vi "test_advanced_Doppler_filtered.vi"() -> ()   [LabVIEW 2009]
doc: "Copyright (C) 2009, Stepan A. Baranov\nweb: http://www.OCTLab.org/\nemail: stepan@baranov.su"
uses:
  OCTLib.dll
panel:
  out "version":string
  out "name":string
  out "error out":errorcluster
  out "max":dbl
  out "min":dbl
  out "window width radius":i32
  out "window height radius":i32
  out "width":i32
  out "height":i32
  in  "Small/Big":bool
  out "loop #":i32
  out "RSM_STAT time":u32
  out "LabView time":u32
  out "RSM_STAT Array":dbl[][](array[numeric])
  out "LabView Array":dbl[][](array[numeric])
  in  "stop":bool
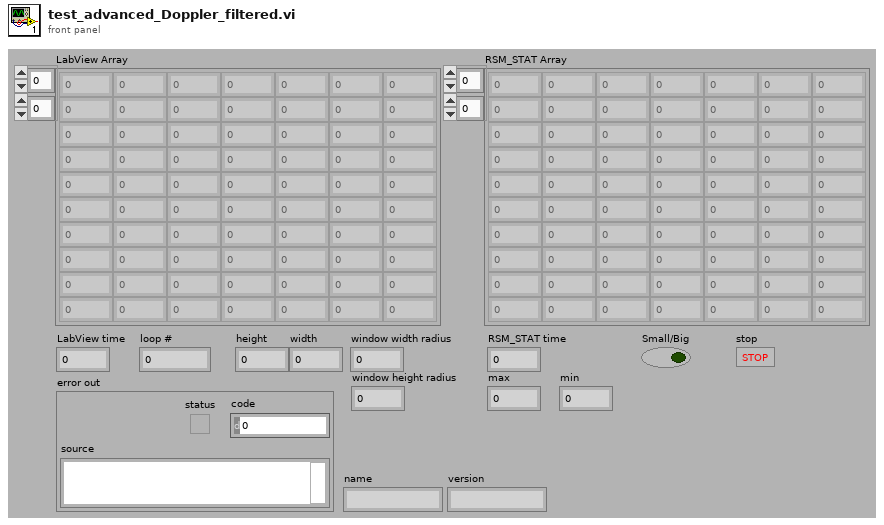
[diagram p1: front panel]
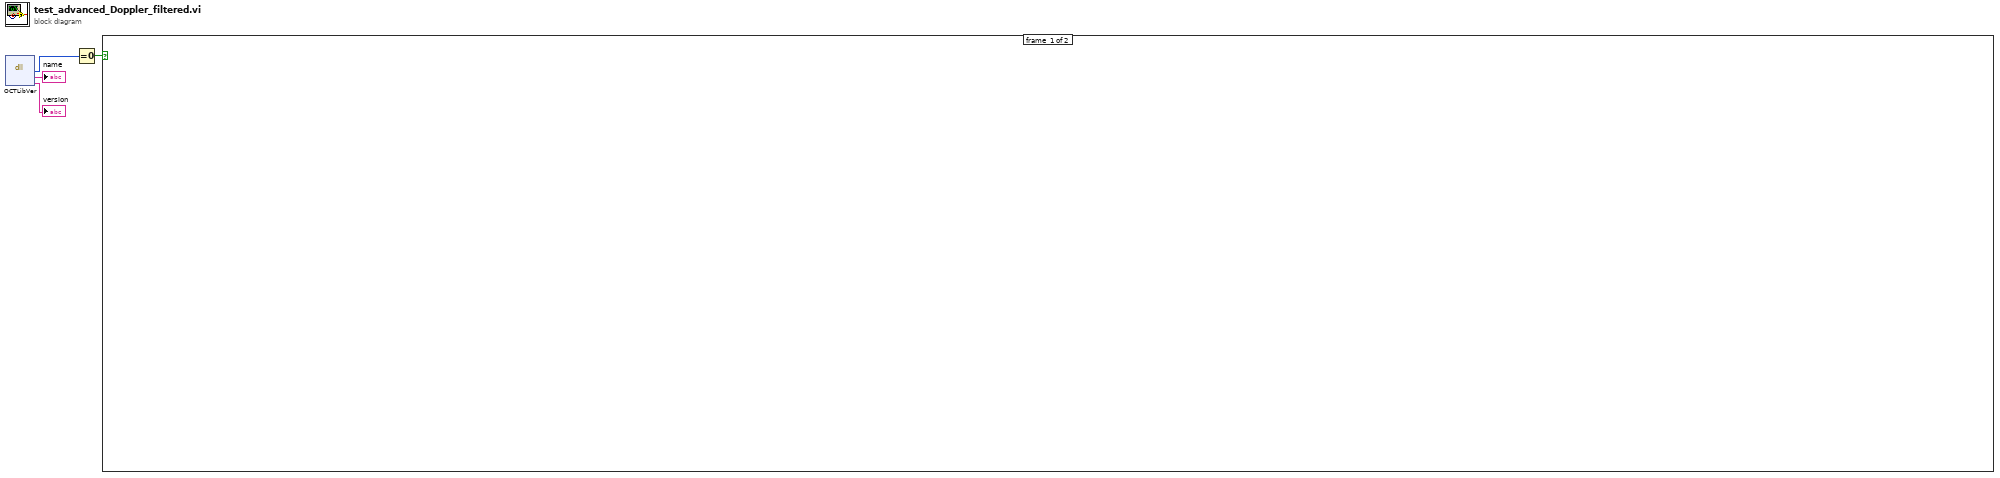
[diagram p0: block diagram]
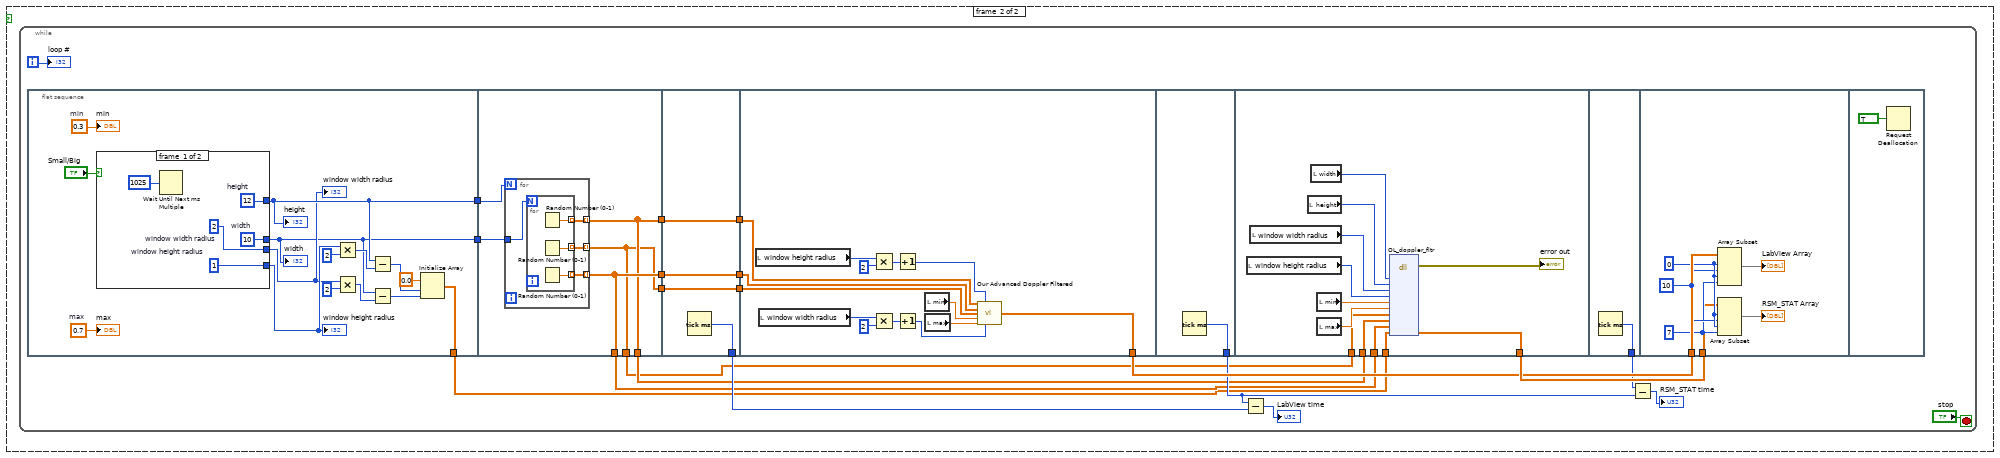
[diagram p2: hidden frame]
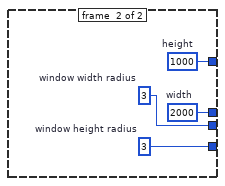
[diagram p3: hidden frame]
diagram:
  n1 = dll-call lib="OCTLib.dll" fn="OCTLibVer"() -> ("status"=w4:i8, "name"=→"name":string, "version"=→"version":string)  [unwired: 5 in, 2 out]
  n2 = Equal To 0?(x=w4) -> (x = 0?=w1:bool)
  n3 = case shown="True" w1 {
    frame #0 {
    }
    frame #1 {
      n4 = while {
        i -> [w17]
        stop <- "stop" stop-if-true
        n5 = flat-sequence {
          tunnel: [w30] -> w13
          tunnel: [w37] -> w12
          tunnel: [w28] -> w8
          tunnel: [w52] -> w16
          tunnel: [w52] -> w14
          tunnel: w13 -> [w54]
          tunnel: w12 -> [w53]
          tunnel: [w51] -> w11
          tunnel: [w51] -> w9
          tunnel: [w50] -> w7
          tunnel: [w50] -> w5
          tunnel: [w65] -> w22
          tunnel: [w64] -> w15
          tunnel: w14 -> [w64]
          tunnel: w11 -> [w62]
          tunnel: [w62] -> w10
          tunnel: w7 -> [w63]
          tunnel: [w63] -> w6
          tunnel: [w71] -> w23
          tunnel: w15 -> [w66]
          tunnel: w10 -> [w68]
          tunnel: w6 -> [w67]
          tunnel: [w80] -> w19
          tunnel: w16 -> [w89]
          tunnel: [w92] -> w24
          tunnel: w9 -> [w88]
          tunnel: w8 -> [w85]
          tunnel: w5 -> [w82]
          tunnel: [w93] -> w20
          tunnel: w24 -> [w94]
          tunnel: w23 -> [w100]
          frame #0 {
            w26 = 0.7  # max
            w27 = 0.3  # min
            n6 = case shown="False" "Small/Big" {
              tunnel: [w44 w49] -> w37
              tunnel: [w45 w48] -> w30
              tunnel: [w42 w47] -> w39
              tunnel: [w41 w46] -> w31
              frame #0 {
                w41 = 2  # window width radius
                w42 = 1  # window height radius
                w45 = 10  # width
                w44 = 12  # height
                n7 = Wait Until Next ms Multiple(millisecond multiple=u32 1025) -> ()  [unwired: 1 out]
              }
              frame #1 {
                w46 = 3  # window width radius
                w47 = 3  # window height radius
                w48 = 2000  # width
                w49 = 1000  # height
              }
            }
            "height" <- w37
            "width" <- w30
            "window height radius" <- w39
            "window width radius" <- w31
            n8 = Multiply(x=w39, y=2) -> (x*y=w36:i32)
            n9 = Multiply(x=w31, y=2) -> (x*y=w32:i32)
            n10 = Subtract(x=w37, y=w36) -> (x-y=w35:i32)
            n11 = Subtract(x=w30, y=w32) -> (x-y=w29:i32)
            n12 = Initialize Array(0.0 ("element"), w35, w29) -> (w28:dbl[][])
            "min" <- w27
            "max" <- w26
          }
          frame #1 {
            n13 = for {
              N: w53 -> [_]
              tunnel: w54 -> [w58]
              tunnel: [w57] -> w52 mode=indexing
              tunnel: [w56] -> w51 mode=indexing
              tunnel: [w55] -> w50 mode=indexing
              n14 = for {
                N: w58 -> [_]
                tunnel: [w61] -> w57 mode=indexing
                tunnel: [w60] -> w56 mode=indexing
                tunnel: [w59] -> w55 mode=indexing
                n15 = Random Number (0-1)() -> (number: 0 to 1=w60:dbl)
                n16 = Random Number (0-1)() -> (number: 0 to 1=w59:dbl)
                n17 = Random Number (0-1)() -> (number: 0 to 1=w61:dbl)
              }
            }
          }
          frame #2 {
            n18 = Tick Count (ms)() -> (millisecond timer value=w65:u32)
          }
          frame #3 {
            n19 = local read "window height radius"() -> (w79:i32)
            n20 = local read "window width radius"() -> (w74:i32)
            n21 = Multiply(x=w79, y=2) -> (x*y=w77:i32)
            n22 = Multiply(x=w74, y=2) -> (x*y=w75:i32)
            n23 = Increment(x=w77) -> (x+1=w72:i32)
            n24 = Increment(x=w75) -> (x+1=w73:i32)
            n25 = local read "min"() -> (w70:dbl)
            n26 = local read "max"() -> (w69:dbl)
            n27 = call "Our Advanced Doppler Filtered.vi"("Real Part"=w68, "Vertical Window"=w72, "Imaginary Part"=w66, "intensity"=w67, "min"=w70, "max"=w69, "Horizontal Window"=w73) -> ("2D Doppler Image"=w71:dbl[][])  [unwired: 8 in]
          }
          frame #4 {
            n28 = Tick Count (ms)() -> (millisecond timer value=w80:u32)
          }
          frame #5 {
            n29 = local read "window height radius"() -> (w86:i32)
            n30 = local read "window width radius"() -> (w87:i32)
            n31 = local read "height"() -> (w90:i32)
            n32 = local read "width"() -> (w91:i32)
            n33 = local read "min"() -> (w83:dbl)
            n34 = local read "max"() -> (w84:dbl)
            n35 = dll-call lib="OCTLib.dll" fn="OL_doppler_fltr"("width"=w91, "height"=w90, "window width radius"=w87, "window height radius"=w86, "min"=w83, "max"=w84, "intensity"=w82, "Re"=w88, "Im"=w89, "data"=w85) -> (error out=→"error out":errorcluster, "data"=w92:dbl[][])  [unwired: 13 in, 1 out]
          }
          frame #6 {
            n36 = Tick Count (ms)() -> (millisecond timer value=w93:u32)
          }
          frame #7 {
            w97 = 10 ("length")
            w96 = 7 ("length")
            w98 = 0 ("index")
            n37 = Array Subset(array=w100, index (row)=w98, length (row)=w97, index (col)=w98, length (col)=w96) -> (→"LabView Array":dbl[][])
            n38 = Array Subset(array=w94, index (row)=w98, length (row)=w97, index (col)=w98, length (col)=w96) -> (→"RSM_STAT Array":dbl[][])
          }
          frame #8 {
            n39 = Request Deallocation(TRUE ("flag")) -> ()
          }
        }
        n40 = Subtract(x=w19, y=w22) -> (x-y=→"LabView time":u32)
        n41 = Subtract(x=w20, y=w19) -> (x-y=→"RSM_STAT time":u32)
        "loop #" <- w17
      }
    }
  }
